vi "get_manifold_pressure.vi"() -> ()   [LabVIEW 2014]
panel:
  in  "stop":bool
  out "standard error":string
  out "standard output":string
  out "text":string
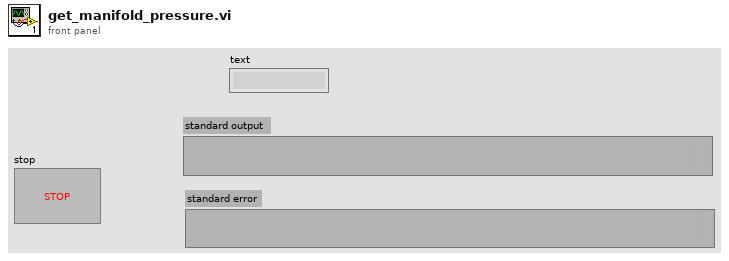
[diagram p1: front panel]
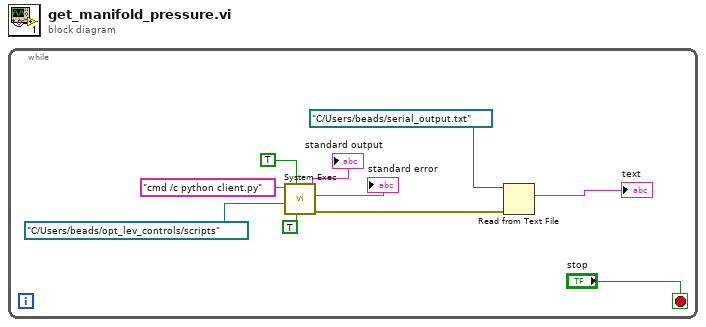
[diagram p0: block diagram]
diagram:
  n1 = while {
    stop <- "stop" stop-if-true
    n2 = call <vilib>:"System Exec.vi"("run minimized? (F)"=TRUE, "wait until completion? (T)"=TRUE, "working directory"=path "C:/Users/beads/opt_lev_controls/scripts", "command line"="cmd /c python client.py") -> ("error out"=w8:errorcluster, "standard error"=→"standard error":string, "standard output"=→"standard output":string)  [unwired: 4 in, 1 out]
    n3 = Read from Text File(file (use dialog)=path "C:/Users/beads/serial_output.txt", error in=w8) -> (text=→"text":string)  [unwired: 2 in, 3 out]
  }
